vi "Actor.vi"(7 "BaseActor":refnum<class "BaseActor.lvclass">, 11 "ErrorQueue":refnum<queue>) -> (4 "Error":errorcluster, 5 "BaseActor":refnum<class "BaseActor.lvclass">)   [LabVIEW 2020, in "jettl.lvlib" / "BaseActor.lvlib" / "BaseActor.lvclass"]
uses:
  BaseActor.lvclass
  BaseActor.lvclass/BaseActor.ctl
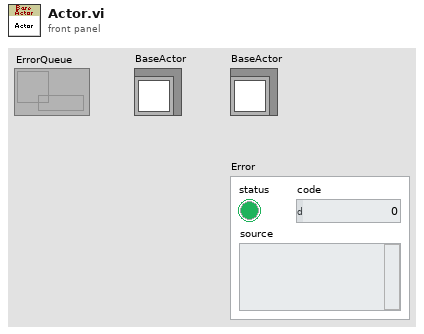
[diagram p1: front panel]
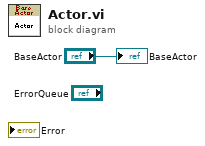
[diagram p0: block diagram]
diagram:
  "BaseActor" <- "BaseActor"
